vi "test5.1-1ToNBroadcastStatus.vi"(8 "error in (no error)":errorcluster, 11 "TestCase in":refnum<class "testcase-CSMBroadcast.lvclass">) -> (0 "error out":errorcluster, 3 "TestCase out":refnum<class "testcase-CSMBroadcast.lvclass">)   [LabVIEW 2017, in "testcase-CSMBroadcast.lvclass"]
uses:
  testcase-CSMBroadcast.lvclass
  0b17d103-e67b-41be-a9eb-a2ee1311ff1f.vi
  5999693e-4f8a-4b34-ae87-f34dff5771be.vi
  src/user.lib/_NEVSTOP/Communicable State Machine(CSM)/AdvanceAPI/CSM - Get Module Attribute.vi
  <vilib>/addons/_JKI Toolkits/VI Tester/TestCase.llb/TestCase.lvclass
  src/user.lib/_NEVSTOP/Communicable State Machine(CSM)/Communicable State Machine.lvlib
  C:/Program Files (x86)/National Instruments/LabVIEW 2017/vi.lib/addons/_JKI Toolkits/VI Tester/TestCase.llb/TestCase.lvclass
panel:
  out "LoopCount2":i32
  out "LoopCount":i32
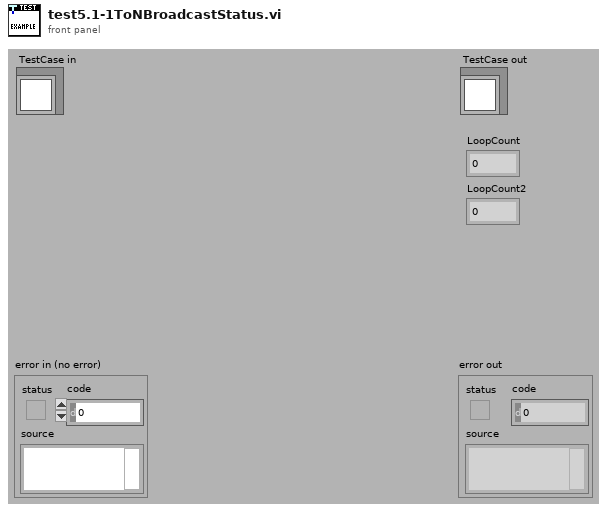
[diagram p1: front panel]
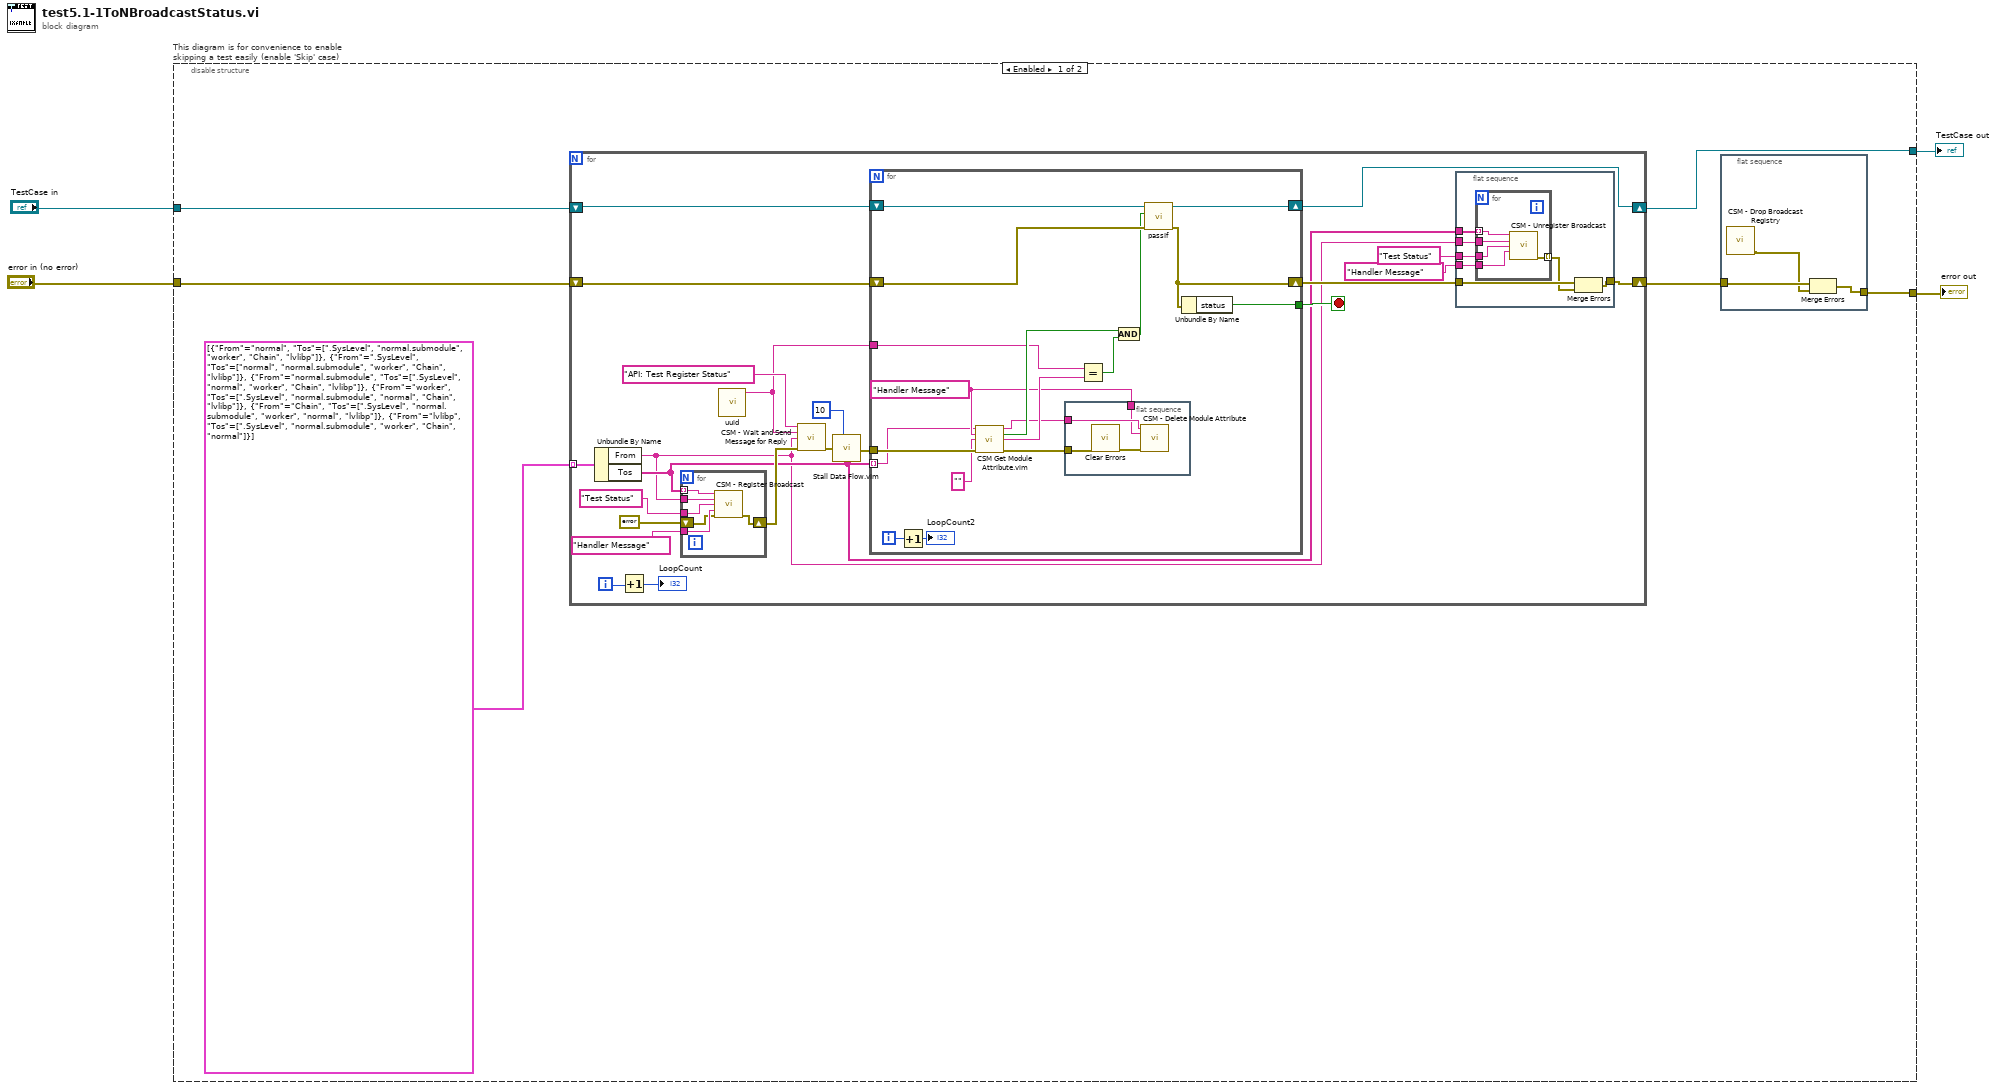
[diagram p0: block diagram]
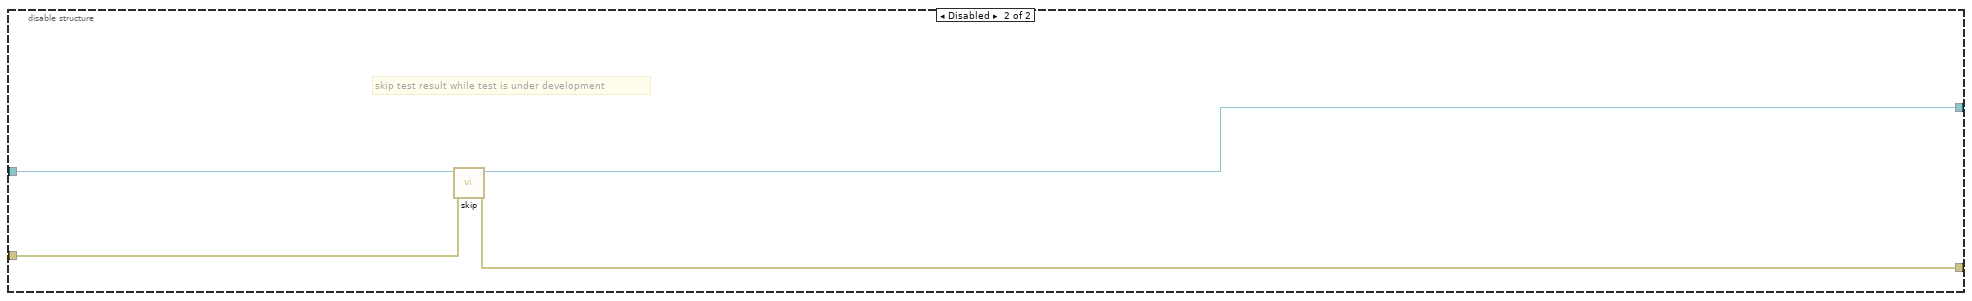
[diagram p2: hidden frame]
diagram:
  n1 = disable-structure "This diagram is for convenience to enable skipping a test easily (enable 'Skip' case)" shown="Enabled" {
    disable-tunnel: "TestCase in" -> [w9 w79]
    disable-tunnel: [w7 w77] -> w1
    disable-tunnel: [w5 w78] -> w3
    disable-tunnel: "error in (no error)" -> [w10 w76]
    frame Enabled {
      n2 = for {
        shift-right: [w19] -> w6
        shift-left: w10 -> [w26]
        shift-right: [w14] -> w7
        shift-left: w9 -> [w27]
        tunnel: cluster{"From":string, "Tos":string[]}[] [{"From"="normal", "Tos"=[".SysLevel", "normal.submodule", "worker", "Chain", "lvlibp"]}, {"From"=".SysLevel", "Tos"=["normal", "normal.submodule", "worker", "Chain", "lvlibp"]}, {"From"="normal.submodule", "Tos"=[".SysLevel", "normal", "worker", "Chain", "lvlibp"]}, {"From"="worker", "Tos"=[".SysLevel", "normal.submodule", "normal", "Chain", "lvlibp"]}, {"From"="Chain", "Tos"=[".SysLevel", "normal.submodule", "worker", "normal", "lvlibp"]}, {"From"="lvlibp", "Tos"=[".SysLevel", "normal.submodule", "worker", "Chain", "normal"]}] -> [w33] mode=indexing
        i -> [w35]
        stop <- w25 stop-if-true
        n3 = Unbundle By Name(w33) -> ("From"=w17:string, "Tos"=w18:string[])
        n4 = Increment(x=w35) -> (x+1=→"LoopCount":i32)
        n5 = for {
          tunnel: w17 -> [w75]
          tunnel: w18 -> [w74] mode=indexing
          tunnel: "Test Status" -> [w73]
          tunnel: "Handler Message" -> [w72]
          shift-right: [w71] -> w21
          shift-left: errorcluster {"status"=FALSE, "code"=0, "source"=""} ("error out") -> [w70]
          n6 = call "CSM - Register Broadcast.vi"("CSM Name(Empty for Broadcast Event)"=w74, "Source CSM Name (* as Default)"=w75, "Trigger"=w73, "API (If \"\", Same as Trigger)"=w72, "Error In"=w70) -> ("error out"=w71:errorcluster)  [unwired: 9 in, 1 out]
        }
        n7 = call "uuid.vi"() -> ("UUID"=w28:string)  [unwired: 11 in]
        n8 = call "CSM - Wait and Send Message for Reply.vi"("State"="API: Test Register Status", "Arguments (\"\")"=w28, "Target Module"=w17, "Error In (No Error)"=w21) -> ("error out"=w31:errorcluster)  [unwired: 9 in, 2 out]
        n9 = call "Stall Data Flow.vim"("value in"=w31, "milliseconds to wait"=u32 10) -> ("value out"=w29:errorcluster)  [unwired: 1 out]
        n10 = for {
          tunnel: w29 -> [w65]
          tunnel: w28 -> [w62]
          tunnel: [w56] -> w25
          shift-right: [w59] -> w14
          shift-left: w27 -> [w60]
          shift-right: [w57] -> w20
          shift-left: w26 -> [w58]
          tunnel: w18 -> [w50] mode=indexing
          i -> [w49]
          w51 = "Handler Message" ("To")
          n11 = Increment(x=w49) -> (x+1=→"LoopCount2":i32)
          n12 = call "CSM Get Module Attribute.vim"("CSM Name"=w50, "Attribute"=w51, "Default Value (Empty Variant)"="", "Error In"=w65) -> ("CSM Name (Dup)"=w52:string, "Found"=w64:bool, "Value"=w61:string, "error out"=w53:errorcluster)  [unwired: 7 in, 1 out]
          n13 = flat-sequence {
            tunnel: w53 -> [w68]
            tunnel: w52 -> [w67]
            tunnel: w51 -> [w66]
            frame #0 {
              n14 = call <vilib>:"Clear Errors.vi"("error in (no error)"=w68) -> ("error out"=w69:errorcluster)  [unwired: 5 in, 1 out]
              n15 = call "CSM - Delete Module Attribute.vi"("CSM Name"=w67, "Attribute"=w66, "Error In"=w69) -> ()  [unwired: 9 in, 4 out]
            }
          }
          n16 = Equal?(x=w62, y=w61) -> (x = y?=w55:bool)
          n17 = And(x=w64, y=w55) -> (x .and. y?=w54:bool)
          n18 = call-dynamic "passIf.vi"("error in (no error)"=w58, "pass"=w54, "TestCase in"=w60) -> ("error out"=w57:errorcluster, "TestCase out"=w59:refnum<class "testcase-CSMBroadcast.lvclass">)  [unwired: 7 in]
          n19 = Unbundle By Name(w57) -> ("status"=w56:bool)
        }
        n20 = flat-sequence {
          tunnel: w20 -> [w41]
          tunnel: [w42] -> w19
          tunnel: w18 -> [w40]
          tunnel: w17 -> [w39]
          tunnel: "Test Status" -> [w38]
          tunnel: "Handler Message" -> [w36]
          frame #0 {
            n21 = for {
              tunnel: w40 -> [w47] mode=indexing
              tunnel: w39 -> [w46]
              tunnel: w38 -> [w45]
              tunnel: [w44] -> w37 mode=indexing
              tunnel: w36 -> [w43]
              n22 = call "CSM - Unregister Broadcast.vi"("CSM Name(Empty for Broadcast Event)"=w47, "Source CSM Name (* as Default)"=w46, "Trigger"=w45, "API (\"*\" as Default)"=w43) -> ("error out"=w44:errorcluster)  [unwired: 10 in, 1 out]
            }
            n23 = Merge Errors(w41, w37) -> (w42:errorcluster)
          }
        }
      }
      n24 = flat-sequence {
        tunnel: [w13] -> w5
        tunnel: w6 -> [w12]
        frame #0 {
          n25 = call "CSM - Drop Broadcast Registry.vi"() -> ("error out"=w11:errorcluster)  [unwired: 15 in]
          n26 = Merge Errors(w12, w11) -> (w13:errorcluster)
        }
      }
    }
    frame Disabled {
      # "skip test result while test is under development"
      n27 = call <vilib>:"skip.vi"("error in (no error)"=w76, "TestCase in"=w79) -> ("error out"=w78:errorcluster, "TestCase out"=w77:refnum<class "testcase-CSMBroadcast.lvclass">)  [unwired: 8 in]
    }
  }
  "error out" <- w3
  "TestCase out" <- w1
